vi "PressureFillLevelCtl.vi"(4 "LiquidValve":bool, 5 "GasValve":bool, 6 "FillLevelCtl":bool, 7 "PressureCtl":bool, 8 "V_setpoint":sgl, 9 "V_value":dbl, 10 "P_setpoint":sgl, 11 "P_value":dbl) -> (0 "LiquidValve":bool, 3 "GasValve":bool)   [LabVIEW 2011]
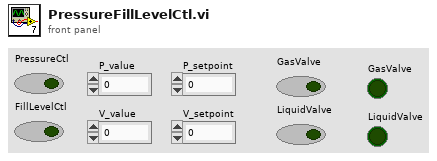
[diagram p1: front panel]
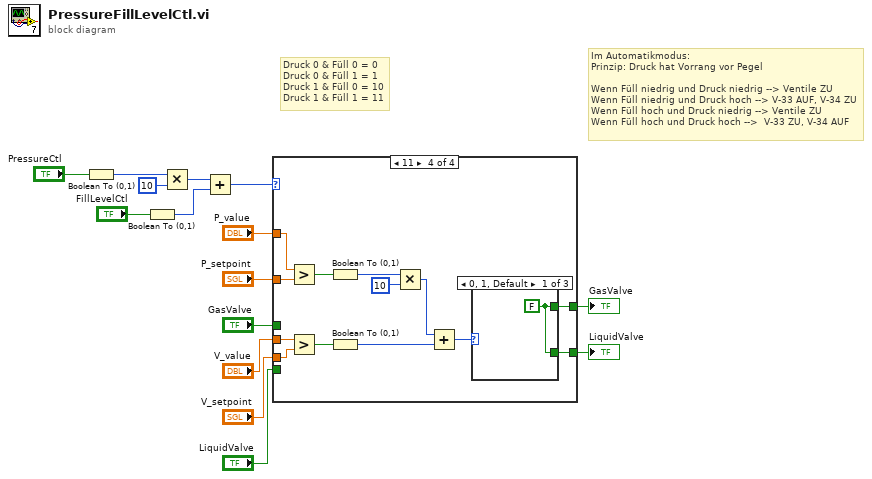
[diagram p0: block diagram]
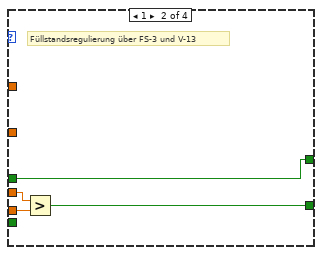
[diagram p3: hidden frame]
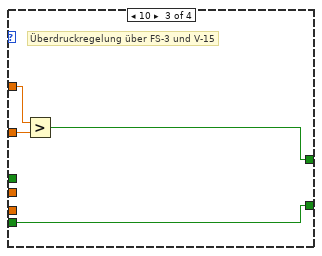
[diagram p4: hidden frame]
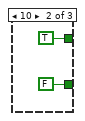
[diagram p5: hidden frame]
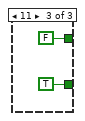
[diagram p6: hidden frame]
diagram:
  # "Im Automatikmodus:\nPrinzip: Druck hat Vorrang vor Pegel\n\nWenn Füll niedrig und Druck niedrig --> Ventile ZU\nWenn Füll niedrig und Druck hoch --> V-33 AUF, V-34 ZU\nWenn Füll hoch und Druck niedrig --> Ventile ZU\nWenn Füll hoch und Druck hoch -->  V-33 ZU, V-34 AUF"
  # "Druck 0 & Füll 0 = 0\nDruck 0 & Füll 1 = 1\nDruck 1 & Füll 0 = 10\nDruck 1 & Füll 1 = 11"
  n1 = Boolean To (0,1)(Boolean="PressureCtl") -> (0, 1=w15:i16)
  n2 = Boolean To (0,1)(Boolean="FillLevelCtl") -> (0, 1=w12:i16)
  n3 = Multiply(x=w15, y=i16 10) -> (x*y=w13:i16)
  n4 = Add(x=w13, y=w12) -> (x+y=w9:i16)
  n5 = case shown="11" w9 {
    tunnel: [w17 w18 w22 w27] -> w8
    tunnel: "GasValve" -> [w17 w18 _ _]
    tunnel: [w16 w19 w23 w26] -> w6
    tunnel: "LiquidValve" -> [w16 _ w23 _]
    tunnel: "P_value" -> [_ _ w25 w31]
    tunnel: "P_setpoint" -> [_ _ w24 w28]
    tunnel: "V_value" -> [_ w20 _ w30]
    tunnel: "V_setpoint" -> [_ w21 _ w29]
    frame 0, Default {
    }
    frame 1 {
      # "Füllstandsregulierung über FS-3 und V-13"
      n6 = Greater?(x=w20, y=w21) -> (0:w19:bool)
    }
    frame 10 {
      # "Überdruckregelung über FS-3 und V-15"
      n7 = Greater?(x=w25, y=w24) -> (0:w22:bool)
    }
    frame 11 {
      n8 = Greater?(x=w31, y=w28) -> (0:w38:bool)
      n9 = Greater?(x=w30, y=w29) -> (0:w37:bool)
      n10 = Boolean To (0,1)(Boolean=w38) -> (0, 1=w34:i16)
      n11 = Boolean To (0,1)(Boolean=w37) -> (0, 1=w36:i16)
      n12 = Multiply(x=w34, y=i16 10) -> (x*y=w32:i16)
      n13 = Add(x=w32, y=w36) -> (x+y=w35:i16)
      n14 = case shown="0, 1, Default" w35 {
        tunnel: [w39 TRUE ("auto? (T)") FALSE ("auto? (T)")] -> w27
        tunnel: [w39 FALSE ("auto? (T)") TRUE ("auto? (T)")] -> w26
        frame 0, 1, Default {
          w39 = FALSE ("auto? (T)")
        }
        frame 10 {
        }
        frame 11 {
        }
      }
    }
  }
  "GasValve" <- w8
  "LiquidValve" <- w6
